vi "Agilent 3352X Series Modulated Waveform.vi"() -> ()   [LabVIEW 2013]
doc: "Shows how to configure and generate an amplitude modulated waveform.\nThe Carrier waveform function is limited by modulation type. (Refer specified modulation VI for detail)"
uses:
  Agilent 3352X Series.lvlib
  Public/Configure/Modulation/Configure Modulation (Amplitude).vi
panel:
  in  "Modulation Function (0: Sine)":u16(ring) items=["Sine", "Square", "Ramp", "NRamp", "Triangle", "Noise", "PRBS", "ARB"]
  in  "AM Source (0: Internal)":u16(ring) items=["Internal", "External", "CH1", "CH2"]
  in  "Modulation Frequency/Sample Rate (100 Hz)":dbl=100.0 format="%#.4f"
  in  "Modulation Depth (100 Percent)":dbl=100.0
  in  "DC Offset (0 V)":dbl
  in  "Frequency/Sample Rate/Bandwidth (1000 Hz)":dbl=1000.0 format="%#.4f"
  in  "Waveform Function (0: Sine)":u16(ring) items=["Sine"=0, "Square"=1, "Ramp"=2, "Noise"=3, "DC"=4, "Triangle"=5, "Pulse"=6, "Sinc"=11, "D-Lorentz"=12, "Gaussian"=13, "Expo Fall"=14, "Expo Rise"=15, "Haversine"=16]
  in  "Amplitude (0.1 Vpp)":dbl=0.1
  in  "VISA resource name":refnum<visa-resource-name>
  # "(c) 2011-2021 National Instruments.  ALL RIGHTS RESERVED."
  # "Carrier Settings"
  # "Modulation Settings"
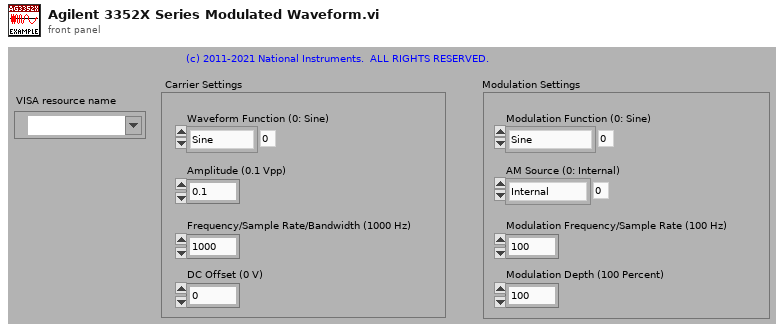
[diagram p1: front panel]
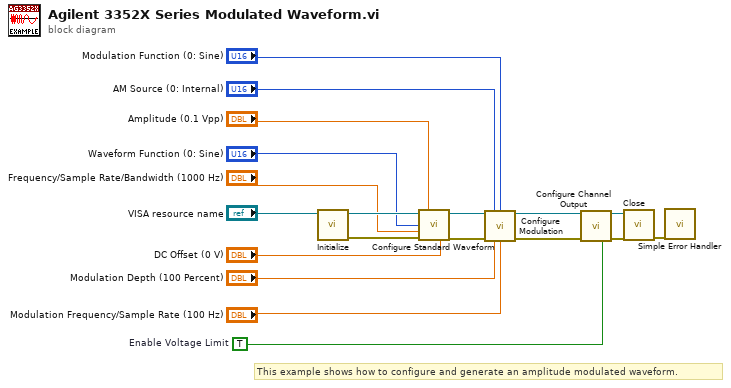
[diagram p0: block diagram]
diagram:
  w12 = TRUE  # Enable Voltage Limit
  # "This example shows how to configure and generate an amplitude modulated waveform."
  n1 = call "Initialize.vi"("VISA resource name"="VISA resource name") -> ("error out"=w17:errorcluster, "VISA resource name out"=w19:refnum<visa-resource-name>)  [unwired: 3 in, 6 out]
  n2 = call "Configure Standard Waveform.vi"("VISA resource name"=w19, "Amplitude (0.1 Vpp)"="Amplitude (0.1 Vpp)", "Waveform Function (0: Sine)"="Waveform Function (0: Sine)", "Frequency/Sample Rate/Bandwidth (1000 Hz)"="Frequency/Sample Rate/Bandwidth (1000 Hz)", "error in (no error)"=w17, "DC Offset (0 V)"="DC Offset (0 V)") -> ("VISA resource name out"=w16:refnum<visa-resource-name>, "error out"=w15:errorcluster)  [unwired: 4 in, 4 out]
  n3 = call-poly "Configure Modulation.vi"("VISA resource name"=w16, "AM Source (0: Internal)"="AM Source (0: Internal)", "Modulation Function (0: Sine)"="Modulation Function (0: Sine)", "error in (no error)"=w15, "Modulation Depth (100 Percent)"="Modulation Depth (100 Percent)", "Modulation Frequency (100 Hz)"="Modulation Frequency/Sample Rate (100 Hz)") -> ("VISA resource name out"=w14:refnum<visa-resource-name>, "error out"=w13:errorcluster)  [unwired: 4 in, 4 out]
  n4 = call "Configure Channel Output.vi"("VISA resource name"=w14, "error in (no error)"=w13, "Enable Voltage Limit (T: Enable)"=w12) -> ("VISA resource name out"=w11:refnum<visa-resource-name>, "error out"=w10:errorcluster)  [unwired: 7 in, 4 out]
  n5 = call "Close.vi"("error in (no error)"=w10, "VISA resource name"=w11) -> ("error out"=w9:errorcluster)  [unwired: 9 out]
  n6 = call <vilib>:"Simple Error Handler.vi"("error in (no error)"=w9) -> ()  [unwired: 1 in, 8 out]
